vi "qrpostion.vi"() -> ()   [LabVIEW 2019]
uses:
  <vilib>/vision/Instrument.llb/QR Code Report.ctl
  <vilib>/vision/Instrument.llb/QR Code Model Type.ctl
  <vilib>/vision/Instrument.llb/QR Code Stream Mode Type.ctl
  <vilib>/vision/Instrument.llb/Data Matrix Polarity.ctl
  <vilib>/vision/Instrument.llb/Demodulation Mode.ctl
  <vilib>/vision/Instrument.llb/Cell Sample Size.ctl
  <vilib>/vision/Instrument.llb/Cell Filter Mode.ctl
panel:
  out "x-y":dbl
  out "Array":string[][](array[string])
  out "Data":string
  out "QR Barcode Report (2D Barcode Reader 1)":T1={"Found?"=FALSE, "Data"="", "Bounding Box"=[], "Errors Corrected"=0, "Dimensions (Rows/Cols)"=0, "Version"=0, "QR Model"=3, "Stream Mode"=0, "Barcode Polarity"=-2, "Mirrored?"=FALSE, "Append Stream Position"=0, "Size of Append Stream"=0, "First EAN-128 ID"=0, "First Alternate Language ID"=0, "Append Stream ID"=0, "Minimum Edge Strength"=30, "Demodulation Mode"=-2, "Cell Sample Size"=-2, "Cell Filter Mode"=-2} {"Append Stream ID" format="%x"; "Cell Filter Mode" items=["Auto-detect"=-2, "Average"=0, "Median"=1, "Central Average"=2, "High Average"=3, "Low Average"=4, "Very High Average"=5, "Very Low Average"=6, "All Filters"=8]; "Cell Sample Size" items=["Auto-detect"=-2, "1x1"=1, "2x2"=2, "3x3"=3, "4x4"=4, "5x5"=5, "6x6"=6, "7x7"=7]; "Demodulation Mode" items=["Auto-detect"=-2, "Histogram"=0, "Local Contrast"=1, "Combination"=2, "All"=3]; "Barcode Polarity" items=["Auto-detect"=-2, "Black on White"=0, "White on Black"=1]; "Stream Mode" items=["Auto-detect", "Numeric", "AlphaNumeric", "Mixed", "Raw Bytes", "UCC/EAN-128 - In Tokens", "UCC/EAN-128 - In Data", "Extended Character Interpretation", "Kanji"]; "QR Model" items=["Auto Detect", "Micro", "Model 1", "Model 2"]; "Version" max=40 step=1}
  out "Ry":i32
  out "Ly":i32
  out "Rx":dbl
  out "Lx":dbl
  in  "Numeric 2":dbl
  in  "Numeric":dbl
  in  "Stop (F)":bool
  out "Image Out":T8(plugin-control)
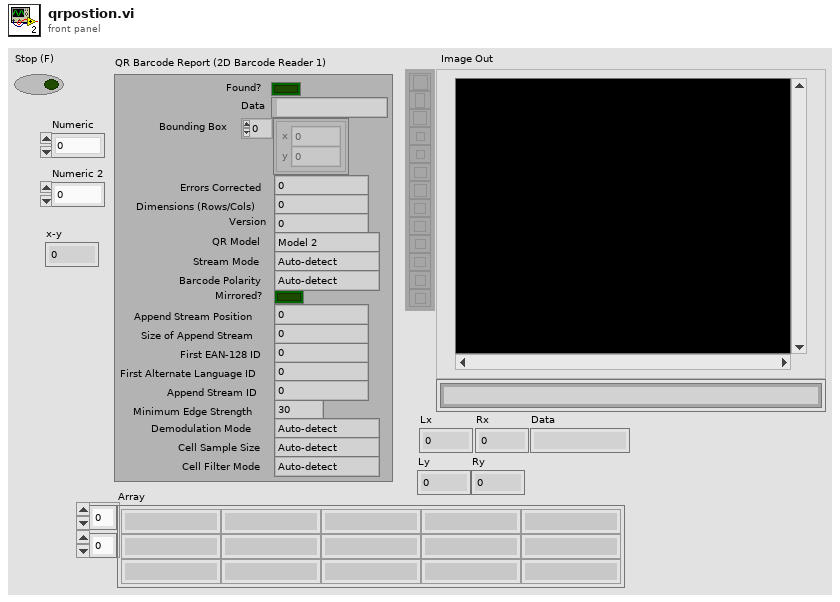
[diagram p1: front panel]
types:
  T1 = typedef "QR Code Report.ctl" = cluster{"Found?":bool, "Data":string, "Bounding Box":cluster{"x":sgl, "y":sgl}[], "Errors Corrected":u32, "Dimensions (Rows/Cols)":u32, "Version":u32, "QR Model":T2, "Stream Mode":T3, "Barcode Polarity":T4, "Mirrored?":bool, "Append Stream Position":u32, "Size of Append Stream":u32, "First EAN-128 ID":i32, "First Alternate Language ID":i32, "Append Stream ID":u32, "Minimum Edge Strength":u32, "Demodulation Mode":T5, "Cell Sample Size":T6, "Cell Filter Mode":T7}
  T2 = typedef "QR Code Model Type.ctl" = i32
  T3 = typedef "QR Code Stream Mode Type.ctl" = i32
  T4 = typedef "Data Matrix Polarity.ctl" = i32
  T5 = typedef "Demodulation Mode.ctl" = i32
  T6 = typedef "Cell Sample Size.ctl" = i32
  T7 = typedef "Cell Filter Mode.ctl" = i32
  T8 = typedef "IMAQ Image.ctl" = refnum<image>
  T9 = typedef "ROI Descriptor" = cluster{"Global Rectangle":i32[], "Contours":cluster{"ID":enum32{"External", "Internal"}, "Type":u32, "Coordinates":i32[]}[]}
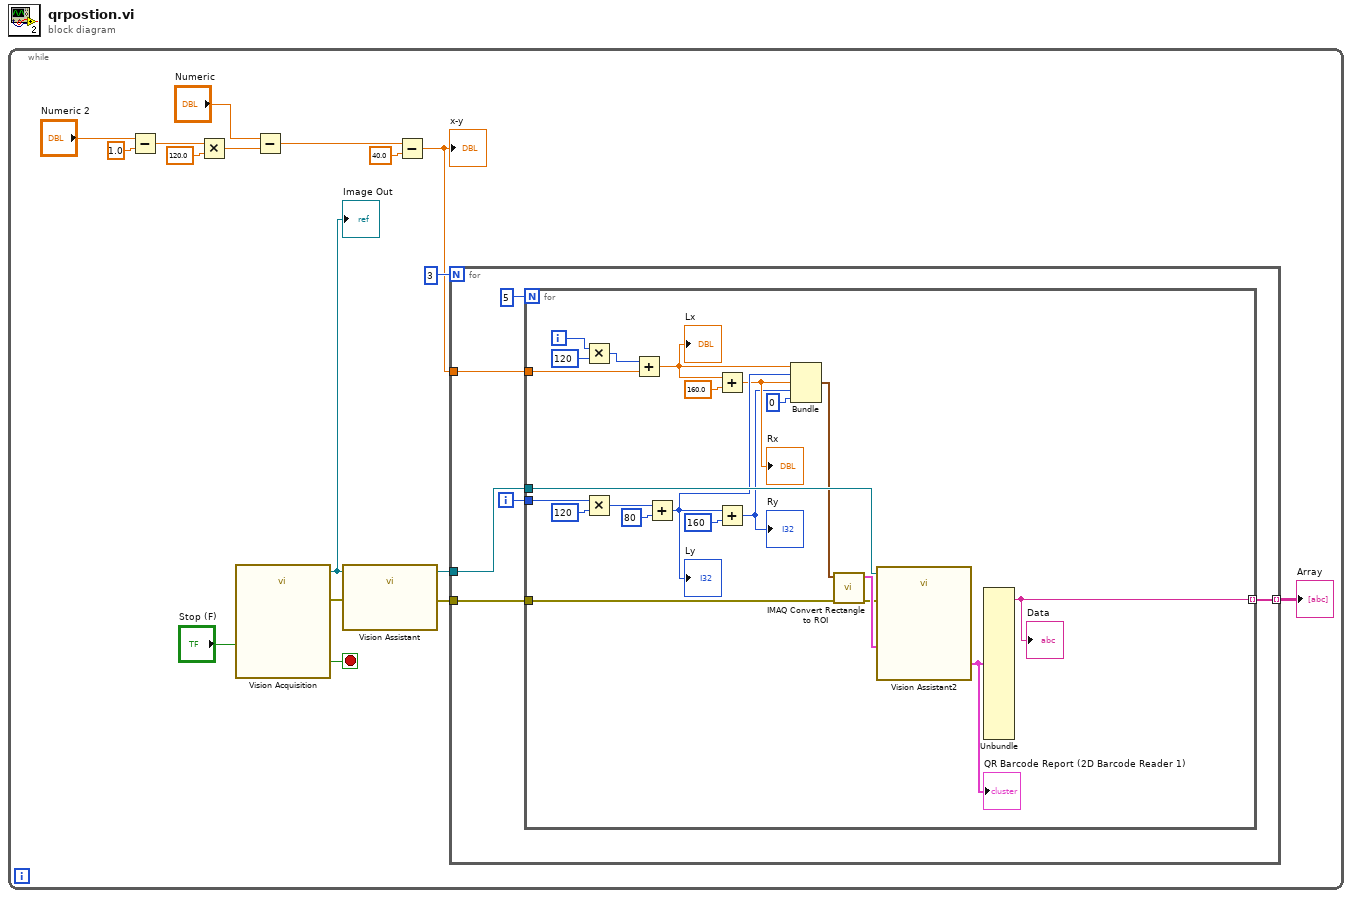
[diagram p0: block diagram]
diagram:
  n1 = while {
    stop <- w16 stop-if-true
    n2 = Subtract(x="Numeric 2", y=1.0) -> (x-y=w12:dbl)
    n3 = Multiply(x=w12, y=120.0) -> (x*y=w1:dbl)
    n4 = call "Vision Acquisition"("Stop (F)"="Stop (F)") -> ("Image Out"=w15:T8, "Stopped"=w16:bool, "error out"=w5:errorcluster)  [unwired: 24 in]
    "Image Out" <- w15
    n5 = Subtract(x="Numeric", y=w1) -> (x-y=w9:dbl)
    n6 = call "Vision Assistant"("Image In"=w15, "error in"=w5) -> ("Image Out"=w13:T8, "error out"=w6:errorcluster)  [unwired: 24 in]
    n7 = Subtract(x=w9, y=40.0) -> (x-y=w7:dbl)
    "x-y" <- w7
    n8 = for {
      N: 3 -> [_]
      tunnel: w13 -> [w22]
      tunnel: w7 -> [w20]
      tunnel: w6 -> [w19]
      tunnel: [w18] -> w4 mode=indexing
      i -> [w21]
      n9 = for {
        N: 5 -> [_]
        tunnel: w22 -> [w45]
        tunnel: w21 -> [w24]
        tunnel: w20 -> [w41]
        tunnel: w19 -> [w28]
        tunnel: [w26] -> w18 mode=indexing
        i -> [w25]
        n10 = Multiply(x=w25, y=120) -> (x*y=w42:i32)
        n11 = Multiply(x=w24, y=120) -> (x*y=w39:i32)
        n12 = Add(x=w42, y=w41) -> (x+y=w35:dbl)
        "Lx" <- w35
        n13 = Add(x=w39, y=80) -> (x+y=w34:i32)
        "Ly" <- w34
        n14 = Add(x=w35, y=160.0) -> (x+y=w33:dbl)
        "Rx" <- w33
        n15 = Add(x=w34, y=160) -> (x+y=w32:i32)
        "Ry" <- w32
        n16 = Bundle(w35, w34, w33, w32, 0) -> (w30:cluster{dbl, i32, dbl, i32, i32})  [unwired: 1 in]
        n17 = call "IMAQ Convert Rectangle to ROI"("error in (no error)"=w28, "Rectangle"=w30) -> ("error out"=w29:errorcluster, "ROI Descriptor"=w44:T9)  [unwired: 7 in]
        n18 = call "Vision Assistant2"("Image In"=w45, "ROI Descriptor (2D Barcode Reader 1)"=w44, "error in"=w29) -> ("QR Barcode Report (2D Barcode Reader 1)"=w27:T1)  [unwired: 22 in, 2 out]
        "QR Barcode Report (2D Barcode Reader 1)" <- w27
        n19 = Unbundle(w27) -> ("Data"=w26:string)  [unwired: 18 out]
        "Data" <- w26
      }
    }
    "Array" <- w4
  }
